vi "DOWNLOAD LOGIC.vi"(7 "Product List":string[][](array[string]), 8 "error in (no error)":errorcluster, 9 "DATA":i64[][](array[numeric])) -> (0 "error out":errorcluster, 1 "product count":i32[][](array[numeric]), 2 "recipe name":i64[][](array[numeric]), 3 "DAy,month,year,hours,minute":i64[][](array[numeric]), 4 "recipe names":string[][](array[string]))   [LabVIEW 2017]
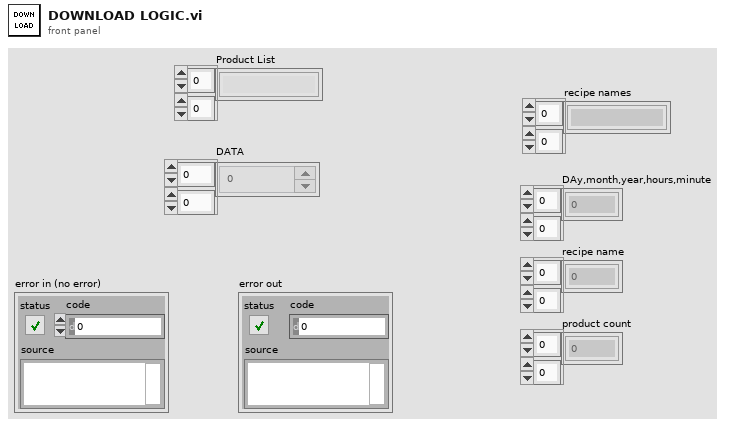
[diagram p1: front panel]
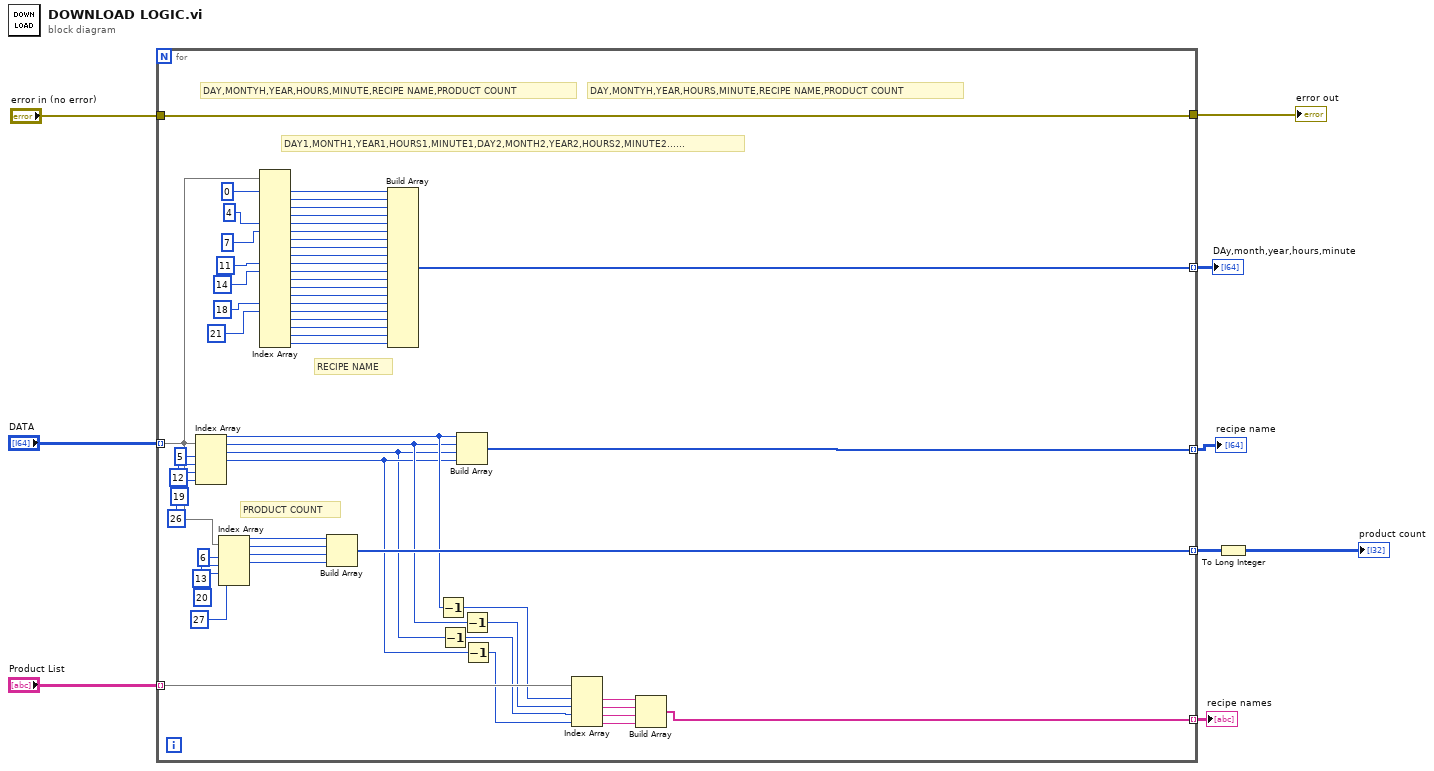
[diagram p0: block diagram]
diagram:
  n1 = for {
    tunnel: [w67] -> w8
    tunnel: "error in (no error)" -> [w67]
    tunnel: "DATA" -> [w47] mode=indexing
    tunnel: [w62] -> w5 mode=indexing
    tunnel: [w53] -> w1 mode=indexing
    tunnel: [w46] -> w6 mode=indexing
    tunnel: "Product List" -> [w23] mode=indexing
    tunnel: [w10] -> w3 mode=indexing
    # "DAY1,MONTH1,YEAR1,HOURS1,MINUTE1,DAY2,MONTH2,YEAR2,HOURS2,MINUTE2......"
    # "PRODUCT COUNT"
    # "RECIPE NAME"
    # "DAY,MONTYH,YEAR,HOURS,MINUTE,RECIPE NAME,PRODUCT COUNT"
    # "DAY,MONTYH,YEAR,HOURS,MINUTE,RECIPE NAME,PRODUCT COUNT"
    n2 = Index Array(array=w47, index #1=5 ("index"), index #2=12 ("index"), index #3=19 ("index"), index #4=26 ("index")) -> (element #1=w21:i64, element #2=w20:i64, element #3=w15:i64, element #4=w16:i64)
    n3 = Index Array(array=w47, index #1=6 ("index"), index #2=13 ("index"), index #3=20 ("index"), index #4=27 ("index")) -> (element #1=w58:i64, element #2=w59:i64, element #3=w60:i64, element #4=w61:i64)
    n4 = Index Array(array=w47, index #1=0 ("index"), index #5=4 ("index"), index #6=7 ("index"), index #10=11 ("index"), index #11=14 ("index"), index #15=18 ("index"), index #16=21 ("index")) -> (element #1=w51:i64, element #2=w50:i64, element #3=w49:i64, element #4=w48:i64, element #5=w39:i64, element #6=w38:i64, element #7=w37:i64, element #8=w36:i64, element #9=w35:i64, element #10=w34:i64, element #11=w33:i64, element #12=w32:i64, element #13=w31:i64, element #14=w30:i64, element #15=w29:i64, element #16=w28:i64, element #17=w27:i64, element #18=w26:i64, element #19=w25:i64, element #20=w24:i64)  [unwired: 13 in]
    n5 = Build Array(w58, w59, w60, w61) -> (w53:i64[])
    n6 = Build Array(w51, w50, w49, w48, w39, w38, w37, w36, w35, w34, w33, w32, w31, w30, w29, w28, w27, w26, w25, w24) -> (w46:i64[])
    n7 = Decrement(x=w21) -> (x-1=w22:i64)
    n8 = Decrement(x=w15) -> (x-1=w18:i64)
    n9 = Build Array(w21, w20, w15, w16) -> (w62:i64[])
    n10 = Decrement(x=w20) -> (x-1=w19:i64)
    n11 = Decrement(x=w16) -> (x-1=w17:i64)
    n12 = Index Array(array=w23, index #1=w22, index #2=w19, index #3=w18, index #4=w17) -> (element #1=w14:string, element #2=w13:string, element #3=w12:string, element #4=w11:string)
    n13 = Build Array(w14, w13, w12, w11) -> (w10:string[])
  }
  "error out" <- w8
  "DAy,month,year,hours,minute" <- w6
  "recipe name" <- w5
  "recipe names" <- w3
  n14 = To Long Integer(number=w1) -> (32bit integer=→"product count":i32[][])
